vi "sum waveform.vi"(0 "RF Freq":dbl format="%#_30g", 2 "phase 1":dbl, 3 "phase 2":dbl, 5 "Cant. Freq":dbl, 7 "no. periods":i32, 9 "Max Sampling Rate":dbl, 12 "Amp 1 (w0)":dbl, 14 "Amp 2 (w0 + wc)":dbl) -> (4 "Waveform Graph":waveform(dbl)(graph), 15 "samples":u32)   [LabVIEW 2018]
panel:
  out "dt":dbl
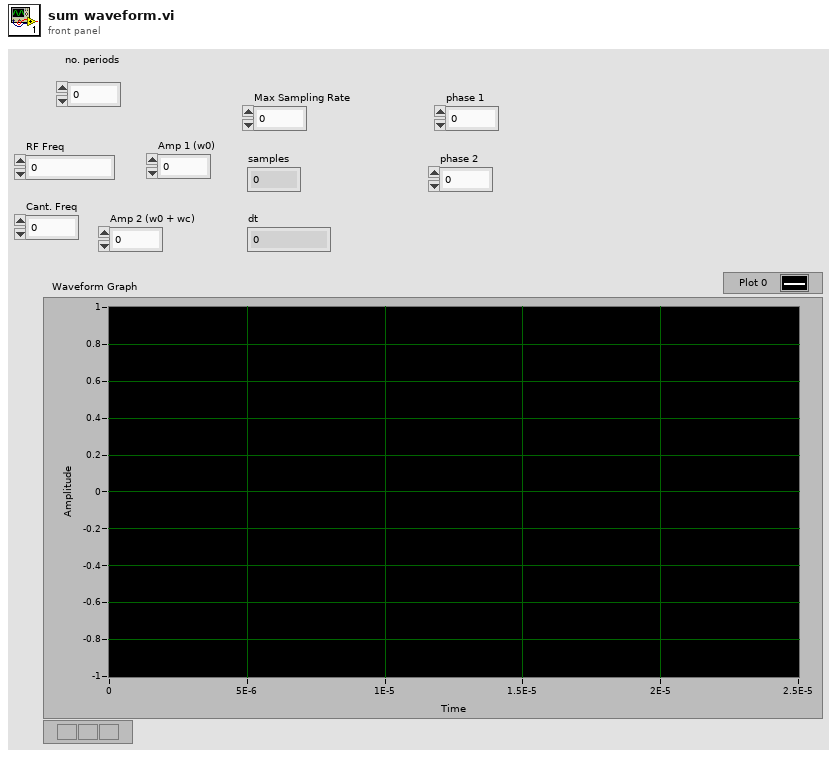
[diagram p1: front panel]
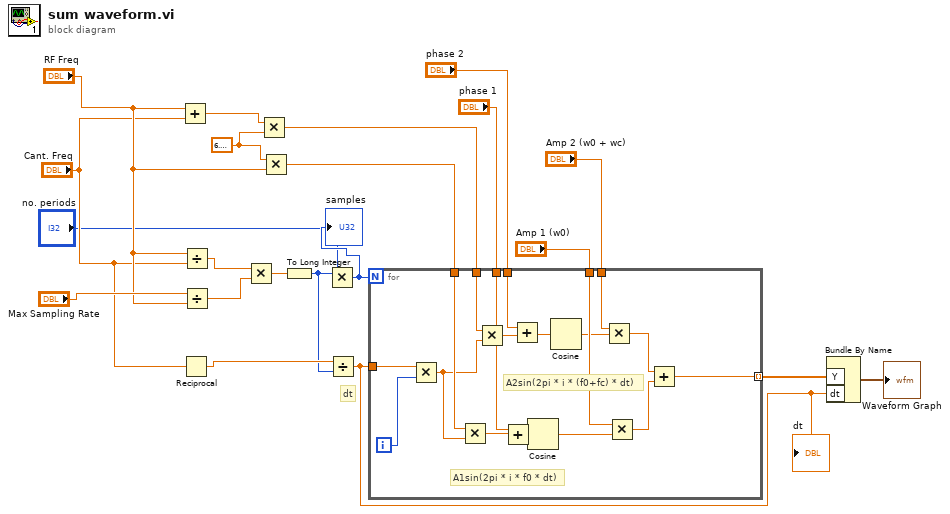
[diagram p0: block diagram]
diagram:
  w20 = 6.283185307179586
  # "dt"
  n1 = Add(x="RF Freq", y="Cant. Freq") -> (x+y=w21:dbl)
  n2 = Reciprocal(x="Cant. Freq") -> (1/x=w16:dbl)
  n3 = Divide(x="RF Freq", y="Cant. Freq") -> (x/y=w18:dbl)
  n4 = Divide(x="Max Sampling Rate", y="RF Freq") -> (x/y=w6:dbl)
  n5 = Multiply(x=w18, y=w6) -> (x*y=w17:dbl)
  n6 = Multiply(x=w21, y=w20) -> (x*y=w15:dbl)
  n7 = Multiply(x=w20, y="RF Freq") -> (x*y=w14:dbl)
  n8 = To Long Integer(number=w17) -> (32bit integer=w3:i32)
  n9 = Multiply(x=w3, y="no. periods") -> (x*y=w2:i32)
  "samples" <- w2
  n10 = Divide(x=w16, y=w3) -> (x/y=w10:dbl)
  "dt" <- w10
  n11 = for {
    N: w2 -> [_]
    tunnel: w10 -> [w38]
    tunnel: w15 -> [w37]
    tunnel: w14 -> [w36]
    tunnel: "Amp 2 (w0 + wc)" -> [w34]
    tunnel: "Amp 1 (w0)" -> [w33]
    tunnel: [w28] -> w11 mode=indexing
    tunnel: "phase 2" -> [w25]
    tunnel: "phase 1" -> [w24]
    i -> [w39]
    # "A2sin(2pi * i * (f0+fc) * dt)"
    # "A1sin(2pi * i * f0 * dt)"
    n12 = Multiply(x=w38, y=w39) -> (x*y=w35:dbl)
    n13 = Multiply(x=w36, y=w35) -> (x*y=w23:dbl)
    n14 = Multiply(x=w37, y=w35) -> (x*y=w26:dbl)
    n15 = Add(x=w24, y=w23) -> (x+y=w22:dbl)
    n16 = Add(x=w25, y=w26) -> (x+y=w27:dbl)
    n17 = Cosine(x=w22) -> (cos(x)=w32:dbl)
    n18 = Cosine(x=w27) -> (cos(x)=w31:dbl)
    n19 = Multiply(x=w34, y=w31) -> (x*y=w30:dbl)
    n20 = Multiply(x=w33, y=w32) -> (x*y=w29:dbl)
    n21 = Add(x=w30, y=w29) -> (x+y=w28:dbl)
  }
  n22 = Bundle By Name("Y"=w11, "dt"=w10) -> (→"Waveform Graph":waveform(dbl))  [unwired: 1 in]
